vi "GOLPI Config Panel.vi"(8 "error in":errorcluster, 11 "session in":T2={"adc"={"niScope"={"channel cfg"=[], "sessions"=[], "multi cards"=FALSE, "channels"=0, "type"=enum."n/a", "memory [B/chn]"=0, "ext. clock [Hz]"=0.0, "samples count"=0, "use streaming"=FALSE, "proc setup"={"packet size [smpl]"=0, "current timeout [s]"=0.0, "blk2blk timeout [s]"=0.0, "event time"=timestamp(0 s since 1904-01-01), "temp sampl T [s]"=0.0, "data queue"=refnum, "stop notifier"=refnum, "proc ref"=refnum}, "sample width [B]"=0, "ranges [V]"=[], "trigger setup"={"coupling"=1, "level [V]"=0.0, "slope"=0, "mode"=enum."Immediate"}, "fs [Hz]"=0.0, "bitres [bit]"=0}, "3458A"={"channels"=[], "sync unit"={"VISA"="", "type"=enum."Picotest U6200A"}, "awg unit"={"type"=enum."Agilent 331xxA to 332xxA", "VISA"="", "enable 10MHz ref"=FALSE}, "sync mode"=enum."MASTER-SLAVE, MASTER clocked by TIMER", "streaming mode"=FALSE, "idn mode"=enum."Auto", "sampling mode"=enum."DCV", "Ts [s]"=0.0, "sample memory [B]"=0, "proc setup"={"channel id"=0, "packet size [smpl]"=0, "current timeout [s]"=0.0, "blk2blk timeout [s]"=0.0, "event time"=timestamp(0 s since 1904-01-01), "stop notifier"=refnum, "data queues"=[], "proc refs"=[], "bus semaphore"=refnum}, "sample size [B]"=0, "sample count"=0, "aux data"={"channel id"=0, "valid?"=[], "gain [V]"=[], "timestamp [s]"=[], "Ts [s]"=0.0, "abs timestamp"=timestamp(0 s since 1904-01-01), "t [deg C]"=[]}, "ranges [V]"=[], "aperture [s]"=0.0, "LEVEL trigger"={"edge"=enum."POS", "level [V]"=0.0, "coupling"=enum."DC"}, "trigger mode"=enum."AUTO", "measure temp.?"=FALSE, "disp mesages"=[], "shared bus?"=FALSE, "disable display?"=FALSE, "aper mode"=enum."Manual", "aper rules"=[]}, "dsdll"={"dsdll"={"dsdll path"=path "", "dsdll handle"=[], "output devices"=[], "capture devices"=[]}, "channels"=0, "device id"=0, "channel idns"=[], "proc setup"={"packet size [smpl]"=0, "current timeout [s]"=0.0, "blk2blk timeout [s]"=0.0, "event time"=timestamp(0 s since 1904-01-01), "data queue"=refnum, "stop notifier"=refnum, "proc ref"=refnum}, "samples count"=0, "fs [Hz]"=0.0}, "type"=enum."niScope", "channel idn str"=[], "aux instr idn str"=[], "modified?"=FALSE, "simadc"={"channels"=[], "range [V]"=0.0, "Ts step [s]"=0.0, "time [s]"=0.0, "fs [Hz]"=0.0, "count"=0, "smpl offset"=0, "set count"=0, "bit res"=0}, "force rst?"=FALSE, "exit mode"=enum."Immediate reset", "exit dly"=0.0, "exit tmr"=timestamp(0 s since 1904-01-01), "busy?"=FALSE, "accessed?"=FALSE, "QuADC session"={"channel cfg"=[], "sessions"=[], "multi cards"=FALSE, "channels"=0, "type"=enum."n/a", "memory [B/chn]"=0, "ext. clock [Hz]"=0.0, "samples count"=0, "use streaming"=FALSE, "proc setup"={"packet size [smpl]"=0, "current timeout [s]"=0.0, "blk2blk timeout [s]"=0.0, "event time"=timestamp(0 s since 1904-01-01), "temp sampl T [s]"=0.0, "data queue"=refnum, "stop notifier"=refnum, "proc ref"=refnum}, "sample width [B]"=0, "ranges [V]"=[], "trigger setup"={"coupling"=1, "level [V]"=0.0, "slope"=0, "mode"=enum."Immediate"}, "fs [Hz]"=0.0, "bitres [bit]"=0}}, "sequence"=[], "sequence setup"={"group setups"=[], "average cycles"=0, "range mode"=enum."Keep defaults", "fs mode"=enum."Frequency", "rng even"=0.0, "rng odd"=0.0, "folder"=path "", "name base"="", "meas id"=0, "settle [s]"=0.0}, "golpi"=refnum, "processing setup"={"mode"=enum."Raw", "call after avgs?"=FALSE, "calculate?"=FALSE, "raw mode"={"command"="", "result mode"=enum."Display console output (only Octave)", "res variable"=""}, "QWTB"={"QWTB path"=path "", "alg filter path"="", "alg ids"=[], "alg parameters"=[], "parsed parameters"=[], "selected alg id"="", "selected unc mode"=enum."None", "qwtb mcc"=100, "qwtb timeout"=90, "qwtb covg"=95.0, "qwtb ofs"=0, "qwtb lim data"=0, "multicore"={"jobs folder"=path "", "cores"=0, "max jobs"=0, "mode"=enum."Singlecore"}, "unc once?"=FALSE}}, "corrections"={"transducers"={"channels"=[], "last path"=path ""}, "digitizer"={"last path"=path "", "channel paths"=[], "channel idns"=[], "correction name"="", "channel names"=[], "folders to copy"=[], "channel valid"=[], "correction path"=path "", "correction rel path"="", "rel folders to copy"=[]}}, "assist cfg"={"P"=0, "Q"=0, "rel shift"=0.0, "ref freq"=0.0, "min fs"=0.0, "max fs tol"=0.0, "min int"=0.0, "max int"=0.0, "max err"=0.0, "max timeout"=0.0}} {"corrections"."transducers"."channels"."Phase index" min=1 step=1; "adc"."QuADC session"."trigger setup"."level [V]" format="%.2f"; "adc"."QuADC session"."trigger setup"."coupling" items=["AC"=0, "DC"=1, "HF Reject"=3, "LF Reject"=4, "AC Plus HF Reject"=1001]; "adc"."QuADC session"."channel cfg"."Clock fr. (Hz)" min=0.0 format="%#_9p"; "adc"."QuADC session"."channel cfg"."Number of JJ" min=1; "adc"."QuADC session"."channel cfg"."Range [Vpk]" min=0.0; "adc"."QuADC session"."channel cfg"."Channel" min=0; "adc"."3458A"."channels"."Range [Vpk]" min=0.0; "adc"."niScope"."trigger setup"."level [V]" format="%.2f"; "adc"."niScope"."trigger setup"."coupling" items=["AC"=0, "DC"=1, "HF Reject"=3, "LF Reject"=4, "AC Plus HF Reject"=1001]; "adc"."niScope"."channel cfg"."Range [Vpk]" min=0.0; "adc"."niScope"."channel cfg"."Channel" min=0}) -> (0 "error out":errorcluster, 3 "session out":T2={"adc"={"niScope"={"channel cfg"=[], "sessions"=[], "multi cards"=FALSE, "channels"=0, "type"=enum."n/a", "memory [B/chn]"=0, "ext. clock [Hz]"=0.0, "samples count"=0, "use streaming"=FALSE, "proc setup"={"packet size [smpl]"=0, "current timeout [s]"=0.0, "blk2blk timeout [s]"=0.0, "event time"=timestamp(0 s since 1904-01-01), "temp sampl T [s]"=0.0, "data queue"=refnum, "stop notifier"=refnum, "proc ref"=refnum}, "sample width [B]"=0, "ranges [V]"=[], "trigger setup"={"coupling"=1, "level [V]"=0.0, "slope"=0, "mode"=enum."Immediate"}, "fs [Hz]"=0.0, "bitres [bit]"=0}, "3458A"={"channels"=[], "sync unit"={"VISA"="", "type"=enum."Picotest U6200A"}, "awg unit"={"type"=enum."Agilent 331xxA to 332xxA", "VISA"="", "enable 10MHz ref"=FALSE}, "sync mode"=enum."MASTER-SLAVE, MASTER clocked by TIMER", "streaming mode"=FALSE, "idn mode"=enum."Auto", "sampling mode"=enum."DCV", "Ts [s]"=0.0, "sample memory [B]"=0, "proc setup"={"channel id"=0, "packet size [smpl]"=0, "current timeout [s]"=0.0, "blk2blk timeout [s]"=0.0, "event time"=timestamp(0 s since 1904-01-01), "stop notifier"=refnum, "data queues"=[], "proc refs"=[], "bus semaphore"=refnum}, "sample size [B]"=0, "sample count"=0, "aux data"={"channel id"=0, "valid?"=[], "gain [V]"=[], "timestamp [s]"=[], "Ts [s]"=0.0, "abs timestamp"=timestamp(0 s since 1904-01-01), "t [deg C]"=[]}, "ranges [V]"=[], "aperture [s]"=0.0, "LEVEL trigger"={"edge"=enum."POS", "level [V]"=0.0, "coupling"=enum."DC"}, "trigger mode"=enum."AUTO", "measure temp.?"=FALSE, "disp mesages"=[], "shared bus?"=FALSE, "disable display?"=FALSE, "aper mode"=enum."Manual", "aper rules"=[]}, "dsdll"={"dsdll"={"dsdll path"=path "", "dsdll handle"=[], "output devices"=[], "capture devices"=[]}, "channels"=0, "device id"=0, "channel idns"=[], "proc setup"={"packet size [smpl]"=0, "current timeout [s]"=0.0, "blk2blk timeout [s]"=0.0, "event time"=timestamp(0 s since 1904-01-01), "data queue"=refnum, "stop notifier"=refnum, "proc ref"=refnum}, "samples count"=0, "fs [Hz]"=0.0}, "type"=enum."niScope", "channel idn str"=[], "aux instr idn str"=[], "modified?"=FALSE, "simadc"={"channels"=[], "range [V]"=0.0, "Ts step [s]"=0.0, "time [s]"=0.0, "fs [Hz]"=0.0, "count"=0, "smpl offset"=0, "set count"=0, "bit res"=0}, "force rst?"=FALSE, "exit mode"=enum."Immediate reset", "exit dly"=0.0, "exit tmr"=timestamp(0 s since 1904-01-01), "busy?"=FALSE, "accessed?"=FALSE, "QuADC session"={"channel cfg"=[], "sessions"=[], "multi cards"=FALSE, "channels"=0, "type"=enum."n/a", "memory [B/chn]"=0, "ext. clock [Hz]"=0.0, "samples count"=0, "use streaming"=FALSE, "proc setup"={"packet size [smpl]"=0, "current timeout [s]"=0.0, "blk2blk timeout [s]"=0.0, "event time"=timestamp(0 s since 1904-01-01), "temp sampl T [s]"=0.0, "data queue"=refnum, "stop notifier"=refnum, "proc ref"=refnum}, "sample width [B]"=0, "ranges [V]"=[], "trigger setup"={"coupling"=1, "level [V]"=0.0, "slope"=0, "mode"=enum."Immediate"}, "fs [Hz]"=0.0, "bitres [bit]"=0}}, "sequence"=[], "sequence setup"={"group setups"=[], "average cycles"=0, "range mode"=enum."Keep defaults", "fs mode"=enum."Frequency", "rng even"=0.0, "rng odd"=0.0, "folder"=path "", "name base"="", "meas id"=0, "settle [s]"=0.0}, "golpi"=refnum, "processing setup"={"mode"=enum."Raw", "call after avgs?"=FALSE, "calculate?"=FALSE, "raw mode"={"command"="", "result mode"=enum."Display console output (only Octave)", "res variable"=""}, "QWTB"={"QWTB path"=path "", "alg filter path"="", "alg ids"=[], "alg parameters"=[], "parsed parameters"=[], "selected alg id"="", "selected unc mode"=enum."None", "qwtb mcc"=100, "qwtb timeout"=90, "qwtb covg"=95.0, "qwtb ofs"=0, "qwtb lim data"=0, "multicore"={"jobs folder"=path "", "cores"=0, "max jobs"=0, "mode"=enum."Singlecore"}, "unc once?"=FALSE}}, "corrections"={"transducers"={"channels"=[], "last path"=path ""}, "digitizer"={"last path"=path "", "channel paths"=[], "channel idns"=[], "correction name"="", "channel names"=[], "folders to copy"=[], "channel valid"=[], "correction path"=path "", "correction rel path"="", "rel folders to copy"=[]}}, "assist cfg"={"P"=0, "Q"=0, "rel shift"=0.0, "ref freq"=0.0, "min fs"=0.0, "max fs tol"=0.0, "min int"=0.0, "max int"=0.0, "max err"=0.0, "max timeout"=0.0}} {"corrections"."transducers"."channels"."Phase index" min=1 step=1; "adc"."QuADC session"."trigger setup"."level [V]" format="%.2f"; "adc"."QuADC session"."trigger setup"."coupling" items=["AC"=0, "DC"=1, "HF Reject"=3, "LF Reject"=4, "AC Plus HF Reject"=1001]; "adc"."QuADC session"."channel cfg"."Clock fr. (Hz)" min=0.0 format="%#_9p"; "adc"."QuADC session"."channel cfg"."Number of JJ" min=1; "adc"."QuADC session"."channel cfg"."Range [Vpk]" min=0.0; "adc"."QuADC session"."channel cfg"."Channel" min=0; "adc"."3458A"."channels"."Range [Vpk]" min=0.0; "adc"."niScope"."trigger setup"."level [V]" format="%.2f"; "adc"."niScope"."trigger setup"."coupling" items=["AC"=0, "DC"=1, "HF Reject"=3, "LF Reject"=4, "AC Plus HF Reject"=1001]; "adc"."niScope"."channel cfg"."Range [Vpk]" min=0.0; "adc"."niScope"."channel cfg"."Channel" min=0})   [LabVIEW 2018]
doc: "This is panel for configuration of Octave/Matlab interface."
uses:
  measure/Meas Session.ctl
  adc/ADC Session.ctl
  drivers/niScope/niScope Session.ctl
  drivers/niScope/niScope Virtual Channel Config.ctl
  drivers/niScope/niScope Virtual Channel Mode.ctl
  drivers/niScope/niScope Virtual Channel Input Z.ctl
  drivers/niScope/niScope Virtual Channel Coupling.ctl
  drivers/niScope/niScope Type.ctl
  drivers/niScope/niScope Digitizing Process Options.ctl
  drivers/niScope/niScope Data Packet.ctl
  drivers/niScope/niScope Trigger Setup.ctl
  <instrlib>/niScope/Controls/niScope trigger coupling.ctl
  <instrlib>/niScope/Controls/niScope trigger slope.ctl
  drivers/DMM/3458A Digitizer Session.ctl
  drivers/DMM/3458A Virtual Channel Config.ctl
  drivers/Counter/Counter Session.ctl
  drivers/Counter/Counter Type.ctl
  drivers/AWG/AWG Session.ctl
  drivers/AWG/AWG Type.ctl
  drivers/DMM/3458A Sync Mode.ctl
  drivers/DMM/3458A Idn Mode.ctl
  drivers/DMM/3458A Digitizing Low Levels/Configure/Sampling Mode.ctl
  drivers/DMM/3458A Digitizing Process Options.ctl
  drivers/DMM/3458A Data Packet.ctl
  drivers/DMM/3458A Aux Record Data.ctl
  drivers/DMM/3458A Digitizing Low Levels/Configure/Level Setup.ctl
  drivers/DMM/3458A Digitizing Low Levels/Configure/First Sample Trigger.ctl
  drivers/DMM/3458A Aperture Selection Mode.ctl
  drivers/dsdll/DSDLL Session.ctl
  drivers/dsdll/dsdll source distribution/dsdll_instance.ctl
  drivers/dsdll/dsdll source distribution/dsdll_device_record.ctl
  drivers/dsdll/DSDLL Process Config.ctl
  drivers/dsdll/DSDLL Data Packet.ctl
  adc/ADC Type.ctl
  drivers/simulated_adc/SimAdc Config.ctl
  drivers/simulated_adc/SimAdc Channel Cfg.ctl
  adc/ADC On Close Action.ctl
  drivers/Quatsch_driver/QuADCDriver/QuADC Session.ctl
  drivers/Quatsch_driver/QuADCDriver/QuADC Virtual Channel Config.ctl
  drivers/Quatsch_driver/QuADCDriver/QuADC Virtual Channel Mode.ctl
  drivers/Quatsch_driver/QuADCDriver/QuADC Virtual Channel Input Z.ctl
  drivers/Quatsch_driver/QuADCDriver/QuADC Virtual Channel Coupling.ctl
  drivers/Quatsch_driver/QuADCDriver/QuADC Type.ctl
  drivers/Quatsch_driver/QuADCDriver/QuADC Digitizing Process Options.ctl
  drivers/Quatsch_driver/QuADCDriver/QuADC Data Packet.ctl
  drivers/Quatsch_driver/QuADCDriver/QuADC Trigger Setup.ctl
  measure/Meas Sequence Item.ctl
  measure/Meas Sampling Configuration.ctl
  adc/ADC Trig Config.ctl
  adc/ADC Trig Mode Source.ctl
  adc/ADC Trig Coupling.ctl
  adc/ADC Trig Slope.ctl
  measure/processing/QWTB/Meas Proc QWTB Algorithm Parameter Data.ctl
  measure/Meas Sequence Configuration.ctl
  measure/Meas Range Mode.ctl
  measure/Meas Sampling Rate Mode.ctl
  golpi_session_ref.ctl
  golpi_session.ctl
  GOLPI Library.lvlibp/Public/GOLPI reference Type Def.ctl
  GOLPI Library.lvlibp/LV Process source distribution/Pipe Handle.ctl
  measure/processing/Meas Process Config.ctl
  measure/processing/Meas Process Mode.ctl
  measure/processing/Meas Process Raw Config.ctl
  measure/processing/Meas Process Raw Result Mode.ctl
  measure/processing/QWTB/Meas Proc QWTB Setup.ctl
  measure/processing/QWTB/Meas Proc QWTB Uncertainty Mode.ctl
  measure/processing/QWTB/Meas Proc QWTB Multicore Setup.ctl
  measure/processing/QWTB/Meas Proc QWTB Multicore Type.ctl
  measure/Corrections/Corr Setup.ctl
  measure/Corrections/Corr Tranducer Item.ctl
  measure/Corrections/Corr Digitizers.ctl
  measure/Assist/Assist Panel Setup.ctl
  varilib/SGUI Assign References Mode.ctl
  varilib/SGUI Assign Multiple Strings With Tags By Label.vi
  varilib/varilib.lvlib
  GOLPI Library.lvlibp
  GOLPI Multi Process.lvlib
  GOLPI Library.lvlibp/LV Process source distribution/LV Process library.lvlib
  drivers/niScope/niScope Virtual Digitizer.lvlib
  drivers/DMM/3458A Virtual Digitizer.lvlib
  drivers/Counter/Counter.lvlib
  drivers/AWG/AWG.lvlib
  drivers/DMM/3458A Digitizing Low Levels/3458A Digitizing Low Levels.lvlib
  drivers/dsdll/DSDLL Virtual Digitizer.lvlib
  drivers/Quatsch_driver/QuADCDriver/QuADC Virtual Digitizer.lvlib
  drivers/dsdll/dsdll source distribution/dsdll.lvlib
panel:
  out "golpi":T1
  in  "tc qwtb":enum32{"Page 1", "Page 2"}(tab)
  in  "qwtb filter":string caption="Relative path to the QWTB algorithms filter (list of supported algorithms)"
  out "qwtb status":bool
  in  "btn test qwtb":bool
  in  "qwtb path":path caption="QWTB toolbox root folder path"
  out "qwtb stat str":string caption="Status"
  in  "btn stop":bool
  in  "tc golpi stat":enum32{"Page 1", "Page 2"}(tab)
  out "status":bool
  out "ver":string caption="Octave version"
  in  "btn test":bool
  in  "btn ok":bool
  in  "tc main":enum32{"Page 1", "Page 2"}(tab)
  in  "btn matlab":bool caption="Enable Matlab Script mode"
  in  "btn clr cache":bool caption="Always clear function cache (slower)"
  in  "btn bitstream":bool caption="Use bitstream mode"
  out "golpi stat":bool caption="GOLPI/GNU Octave running?"
  in  "btn console":bool caption="Show console window"
  in  "start timeout [ms]":u32=30000 caption="Startup timeout [ms]"
  in  "octave path":path=path "C:/Octave/Octave_3.6.4/bin" caption="GNU Octave binary path (folder or full path)"
  # "Note: Restart GOLPI to apply changes!"
  # "ADC:"
  # "IP Address"
  # "."
  # "."
  # "."
  # ":"
  # "ADC:"
  # "IP Address"
  # "."
  # "."
  # "."
  # ":"
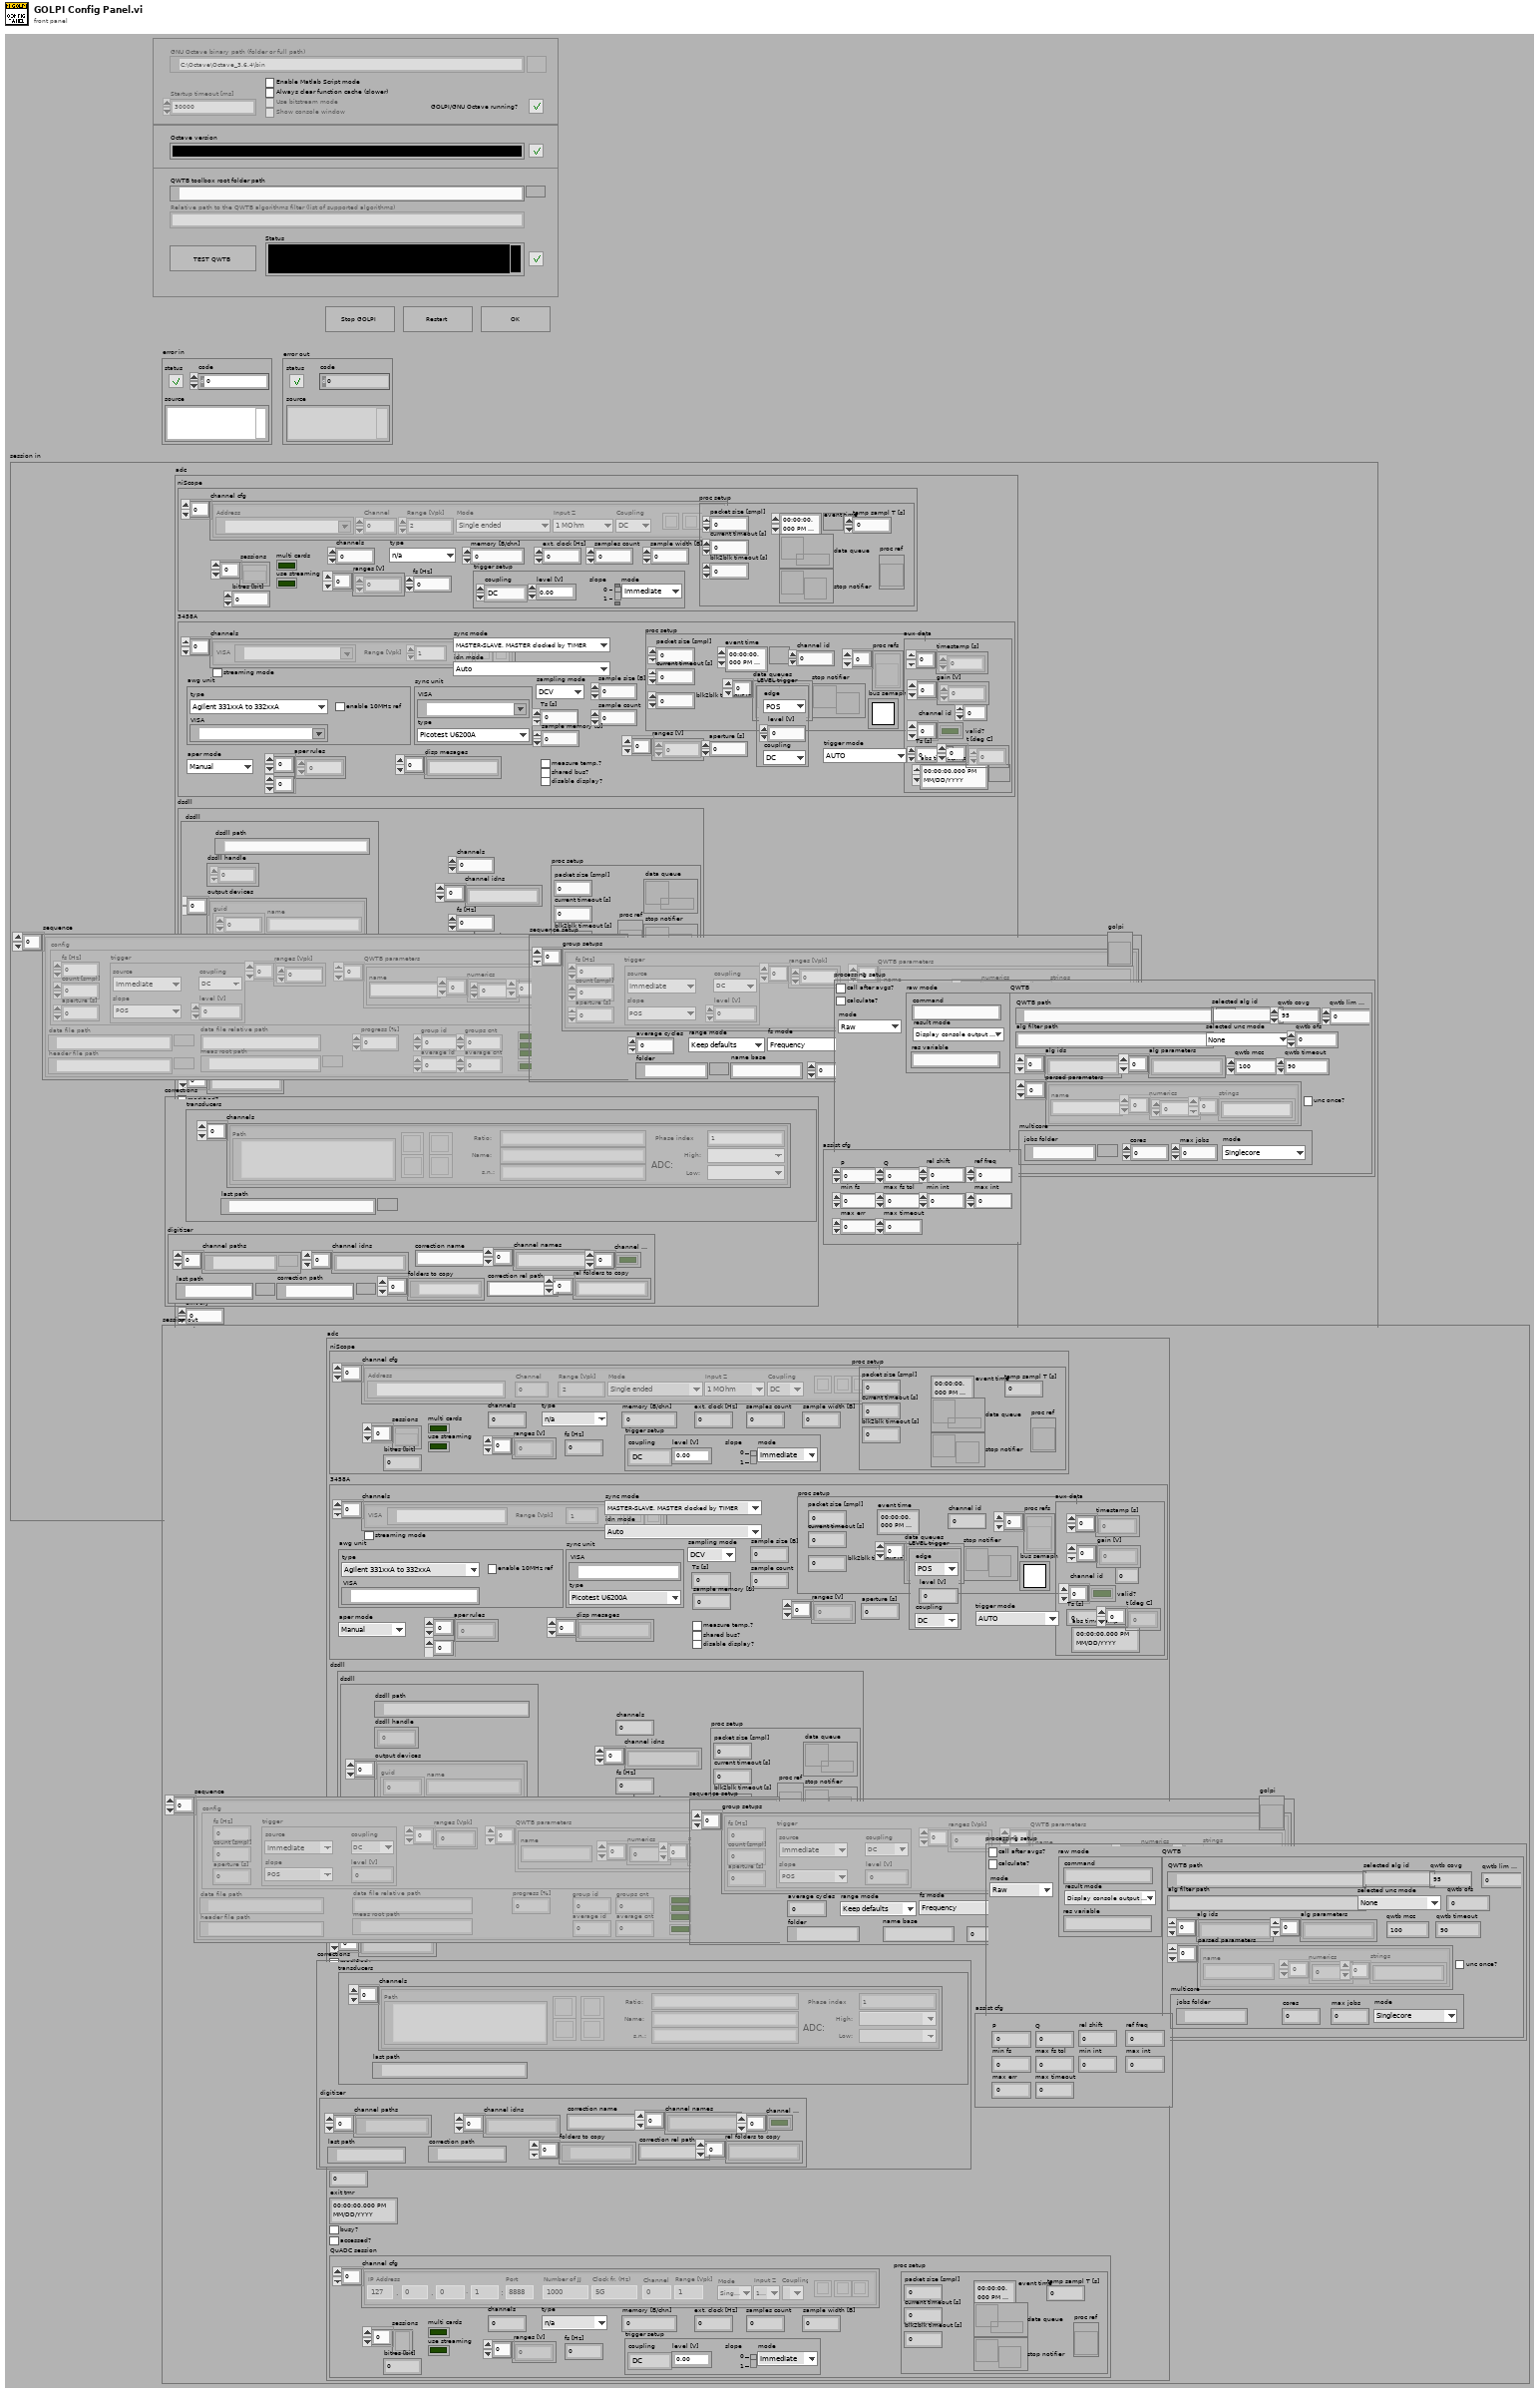
[diagram p1: front panel]
types:
  T1 = typedef "GOLPI Multi Process.lvlib/golpi_session_ref.ctl" = refnum<vi>
  T2 = typedef "Meas Session.ctl" = cluster{"adc":T3, "sequence":T45[], "sequence setup":T52, "golpi":T1, "processing setup":T55, "corrections":T63, "assist cfg":T66}
  T3 = typedef "ADC Session.ctl" = cluster{"niScope":T4, "3458A":T14, "dsdll":T29, "type":T33, "channel idn str":string[], "aux instr idn str":string[], "modified?":bool, "simadc":T34, "force rst?":bool, "exit mode":T36, "exit dly":dbl, "exit tmr":timestamp, "busy?":bool, "accessed?":bool, "QuADC session":T37}
  T4 = typedef "niScope Virtual Digitizer.lvlib/niScope Session.ctl" = cluster{"channel cfg":T5[], "sessions":refnum<k20>[], "multi cards":bool, "channels":i32, "type":T9, "memory [B/chn]":i32, "ext. clock [Hz]":dbl, "samples count":i64, "use streaming":bool, "proc setup":T10, "sample width [B]":i32, "ranges [V]":dbl[], "trigger setup":T11, "fs [Hz]":dbl, "bitres [bit]":i32}
  T5 = typedef "niScope Virtual Digitizer.lvlib/niScope Virtual Channel Config.ctl" = cluster{"Address":refnum<k15>, "Channel":i32, "Mode":T6, "Input Z":T7, "Coupling":T8, "Range [Vpk]":dbl, "btn clr":bool, "btn up":bool, "btn down":bool}
  T6 = typedef "niScope Virtual Digitizer.lvlib/niScope Virtual Channel Mode.ctl" = enum16{"Single ended", "Unbal. differential", "Differential"}
  T7 = typedef "niScope Virtual Digitizer.lvlib/niScope Virtual Channel Input Z.ctl" = enum16{"1 MOhm", "50 Ohm"}
  T8 = typedef "niScope Virtual Digitizer.lvlib/niScope Virtual Channel Coupling.ctl" = enum16{"AC", "DC", "GND"}
  T9 = typedef "niScope Virtual Digitizer.lvlib/niScope Type.ctl" = enum16{"n/a", "5922"}
  T10 = typedef "niScope Virtual Digitizer.lvlib/niScope Digitizing Process Options.ctl" = cluster{"packet size [smpl]":i64, "current timeout [s]":dbl, "blk2blk timeout [s]":dbl, "event time":timestamp, "temp sampl T [s]":dbl, "data queue":refnum<queue>, "stop notifier":refnum<notifier>, "proc ref":refnum<vi>}
  T11 = typedef "niScope Virtual Digitizer.lvlib/niScope Trigger Setup.ctl" = cluster{"coupling":T12, "level [V]":dbl, "slope":T13, "mode":enum16{"Immediate", "External", "Level"}}
  T12 = typedef "niScope trigger coupling.ctl" = u16
  T13 = typedef "niScope trigger slope.ctl" = i32
  T14 = typedef "3458A Virtual Digitizer.lvlib/3458A Digitizer Session.ctl" = cluster{"channels":T15[], "sync unit":T16, "awg unit":T18, "sync mode":T20, "streaming mode":bool, "idn mode":T21, "sampling mode":T22, "Ts [s]":dbl, "sample memory [B]":i32, "proc setup":T23, "sample size [B]":i32, "sample count":i32, "aux data":T25, "ranges [V]":dbl[], "aperture [s]":dbl, "LEVEL trigger":T26, "trigger mode":T27, "measure temp.?":bool, "disp mesages":string[], "shared bus?":bool, "disable display?":bool, "aper mode":T28, "aper rules":dbl[][]}
  T15 = typedef "3458A Virtual Digitizer.lvlib/3458A Virtual Channel Config.ctl" = cluster{"VISA":refnum<visa-resource-name>, "Range [Vpk]":dbl, "btn clr":bool, "btn up":bool, "btn down":bool}
  T16 = typedef "Counter.lvlib/Counter Session.ctl" = cluster{"VISA":refnum<visa-resource-name>, "type":T17}
  T17 = typedef "Counter.lvlib/Counter Type.ctl" = enum16{"Picotest U6200A", "dummy"}
  T18 = typedef "AWG.lvlib/AWG Session.ctl" = cluster{"type":T19, "VISA":refnum<visa-resource-name>, "enable 10MHz ref":bool}
  T19 = typedef "AWG.lvlib/AWG Type.ctl" = enum16{"Agilent 331xxA to 332xxA", "Agilent 335xxA to 336xxA", "Tektronix AFG3101C", "dummy"}
  T20 = typedef "3458A Virtual Digitizer.lvlib/3458A Sync Mode.ctl" = enum16{"MASTER-SLAVE, MASTER clocked by TIMER", "MASTER-SLAVE, MASTER clocked by AWG", "ALL clocked by AWG", "MASTER-SLAVE, ALL clocked by TIMER", "ALL clocked by AWG with DFLL"}
  T21 = typedef "3458A Virtual Digitizer.lvlib/3458A Idn Mode.ctl" = enum16{"Auto", "Sequential (chn A, chn B, ...)", "From calibration string"}
  T22 = typedef "3458A Virtual Digitizer.lvlib/3458A Digitizing Low Levels.lvlib/Sampling Mode.ctl" = enum16{"DCV", "DSDC", "DSAC"}
  T23 = typedef "3458A Virtual Digitizer.lvlib/3458A Digitizing Process Options.ctl" = cluster{"channel id":i32, "packet size [smpl]":i32, "current timeout [s]":dbl, "blk2blk timeout [s]":dbl, "event time":timestamp, "stop notifier":refnum<notifier>, "data queues":refnum<queue>[], "proc refs":refnum<vi>[], "bus semaphore":T24}
  T24 = typedef "Semaphore RefNum" = refnum<k1>
  T25 = typedef "3458A Virtual Digitizer.lvlib/3458A Aux Record Data.ctl" = cluster{"channel id":i32, "valid?":bool[], "gain [V]":dbl[], "timestamp [s]":dbl[], "Ts [s]":dbl, "abs timestamp":timestamp, "t [deg C]":dbl[]}
  T26 = typedef "3458A Virtual Digitizer.lvlib/3458A Digitizing Low Levels.lvlib/Level Setup.ctl" = cluster{"edge":enum16{"POS", "NEG"}, "level [V]":dbl, "coupling":enum16{"DC", "AC"}}
  T27 = typedef "3458A Virtual Digitizer.lvlib/3458A Digitizing Low Levels.lvlib/First Sample Trigger.ctl" = enum16{"AUTO", "EXT", "SYN", "SGL", "HOLD", "LEVEL"}
  T28 = typedef "3458A Virtual Digitizer.lvlib/3458A Aperture Selection Mode.ctl" = enum16{"Manual", "Maximum", "Table"}
  T29 = typedef "DSDLL Virtual Digitizer.lvlib/DSDLL Session.ctl" = cluster{"dsdll":T30, "channels":i32, "device id":i32, "channel idns":string[], "proc setup":T32, "samples count":i32, "fs [Hz]":dbl}
  T30 = typedef "dsdll.lvlib/dsdll_instance.ctl" = cluster{"dsdll path":path, "dsdll handle":u8[], "output devices":T31[], "capture devices":T31[]}
  T31 = typedef "dsdll.lvlib/dsdll_device_record.ctl" = cluster{"guid":u8[], "name":string}
  T32 = typedef "DSDLL Virtual Digitizer.lvlib/DSDLL Process Config.ctl" = cluster{"packet size [smpl]":i32, "current timeout [s]":dbl, "blk2blk timeout [s]":dbl, "event time":timestamp, "data queue":refnum<queue>, "stop notifier":refnum<notifier>, "proc ref":refnum<vi>}
  T33 = typedef "ADC Type.ctl" = enum16{"niScope", "3458A", "DirectSound DLL", "dummy", "QuADC"}
  T34 = typedef "SimAdc Config.ctl" = cluster{"channels":T35[], "range [V]":dbl, "Ts step [s]":dbl, "time [s]":dbl, "fs [Hz]":dbl, "count":i64, "smpl offset":i64, "set count":i64, "bit res":i32}
  T35 = typedef "SimAdc Channel Cfg.ctl" = cluster{"harmonics":dbl[][], "btn clear":bool, "noise":dbl, "fundamental [Hz]":dbl}
  T36 = typedef "ADC On Close Action.ctl" = enum16{"Immediate reset", "Delayed reset"}
  T37 = typedef "QuADC Virtual Digitizer.lvlib/QuADC Session.ctl" = cluster{"channel cfg":T38[], "sessions":refnum<k5>[], "multi cards":bool, "channels":i32, "type":T42, "memory [B/chn]":i32, "ext. clock [Hz]":dbl, "samples count":i64, "use streaming":bool, "proc setup":T43, "sample width [B]":i32, "ranges [V]":dbl[], "trigger setup":T44, "fs [Hz]":dbl, "bitres [bit]":i32}
  T38 = typedef "QuADC Virtual Digitizer.lvlib/QuADC Virtual Channel Config.ctl" = cluster{"Channel":i32, "Mode":T39, "Input Z":T40, "Coupling":T41, "Range [Vpk]":dbl, "btn clr":bool, "btn up":bool, "btn down":bool, "IP address A":u8, "IP address B":u8, "IP address C":u8, "IP address D":u8, "Port":u16, "Number of JJ":u32, "Clock fr. (Hz)":dbl}
  T39 = typedef "QuADC Virtual Digitizer.lvlib/QuADC Virtual Channel Mode.ctl" = enum16{"Single ended", "Unbal. differential", "Differential"}
  T40 = typedef "QuADC Virtual Digitizer.lvlib/QuADC Virtual Channel Input Z.ctl" = enum16{"1 MOhm", "50 Ohm"}
  T41 = typedef "QuADC Virtual Digitizer.lvlib/QuADC Virtual Channel Coupling.ctl" = enum16{"AC", "DC", "GND"}
  T42 = typedef "QuADC Virtual Digitizer.lvlib/QuADC Type.ctl" = enum16{"n/a", "v1"}
  T43 = typedef "QuADC Virtual Digitizer.lvlib/QuADC Digitizing Process Options.ctl" = cluster{"packet size [smpl]":i64, "current timeout [s]":dbl, "blk2blk timeout [s]":dbl, "event time":timestamp, "temp sampl T [s]":dbl, "data queue":refnum<queue>, "stop notifier":refnum<notifier>, "proc ref":refnum<vi>}
  T44 = typedef "QuADC Virtual Digitizer.lvlib/QuADC Trigger Setup.ctl" = cluster{"coupling":T12, "level [V]":dbl, "slope":T13, "mode":enum16{"Immediate", "External", "Level"}}
  T45 = typedef "Meas Sequence Item.ctl" = cluster{"config":T46, "data file path":path, "header file path":path, "group id":i32, "average id":i32, "group done?":bool, "adc modified?":bool, "source modified?":bool, "progress [%]":dbl, "groups cnt":i32, "average cnt":i32, "data file relative path":string, "meas root path":path, "calculate?":bool}
  T46 = typedef "Meas Sampling Configuration.ctl" = cluster{"fs [Hz]":dbl, "count [smpl]":i64, "aperture [s]":dbl, "trigger":T47, "ranges [Vpk]":dbl[], "QWTB parameters":T51[]}
  T47 = typedef "ADC Trig Config.ctl" = cluster{"source":T48, "level [V]":dbl, "coupling":T49, "slope":T50}
  T48 = typedef "ADC Trig Mode Source.ctl" = enum16{"Immediate", "External", "Level"}
  T49 = typedef "ADC Trig Coupling.ctl" = enum16{"DC", "AC"}
  T50 = typedef "ADC Trig Slope.ctl" = enum16{"POS", "NEG"}
  T51 = typedef "Meas Proc QWTB Algorithm Parameter Data.ctl" = cluster{"name":string, "numerics":dbl[], "strings":string[]}
  T52 = typedef "Meas Sequence Configuration.ctl" = cluster{"group setups":T46[], "average cycles":i32, "range mode":T53, "fs mode":T54, "rng even":dbl, "rng odd":dbl, "folder":path, "name base":string, "meas id":i32, "settle [s]":dbl}
  T53 = typedef "Meas Range Mode.ctl" = enum16{"Keep defaults", "Set All channels", "Set Odd and Even channels"}
  T54 = typedef "Meas Sampling Rate Mode.ctl" = enum16{"Frequency", "Period"}
  T55 = typedef "Meas Process Config.ctl" = cluster{"mode":T56, "call after avgs?":bool, "calculate?":bool, "raw mode":T57, "QWTB":T59}
  T56 = typedef "Meas Process Mode.ctl" = enum16{"Raw", "QWTB"}
  T57 = typedef "Meas Process Raw Config.ctl" = cluster{"command":string, "result mode":T58, "res variable":string}
  T58 = typedef "Meas Process Raw Result Mode.ctl" = enum16{"Display console output (only Octave)", "Display string variable", "Display result file %respath%"}
  T59 = typedef "Meas Proc QWTB Setup.ctl" = cluster{"QWTB path":path, "alg filter path":string, "alg ids":string[], "alg parameters":string[], "parsed parameters":T51[], "selected alg id":string, "selected unc mode":T60, "qwtb mcc":i32, "qwtb timeout":i32, "qwtb covg":dbl, "qwtb ofs":i64, "qwtb lim data":i64, "multicore":T61, "unc once?":bool}
  T60 = typedef "Meas Proc QWTB Uncertainty Mode.ctl" = enum16{"None", "GUF", "Monte Carlo"}
  T61 = typedef "Meas Proc QWTB Multicore Setup.ctl" = cluster{"jobs folder":path, "cores":i32, "max jobs":i32, "mode":T62}
  T62 = typedef "Meas Proc QWTB Multicore Type.ctl" = enum16{"Singlecore", "Multicore", "Multistation"}
  T63 = typedef "Corr Setup.ctl" = cluster{"transducers":cluster{"channels":T64[], "last path":path}, "digitizer":T65}
  T64 = typedef "Corr Tranducer Item.ctl" = cluster{"Path":path, "Ratio:":string, "Name:":string, "btn rem":bool, "btn up":bool, "btn down":bool, "s.n.:":string, "btn open":bool, "ratio o/i":dbl, "chn hi":u16, "chn lo":u16, "Phase index":i32}
  T65 = typedef "Corr Digitizers.ctl" = cluster{"last path":path, "channel paths":path[], "channel idns":string[], "correction name":string, "channel names":string[], "folders to copy":path[], "channel valid":bool[], "correction path":path, "correction rel path":string, "rel folders to copy":string[]}
  T66 = typedef "Assist Panel Setup.ctl" = cluster{"P":i32, "Q":i32, "rel shift":dbl, "ref freq":dbl, "min fs":dbl, "max fs tol":dbl, "min int":dbl, "max int":dbl, "max err":dbl, "max timeout":dbl}
  T67 = typedef "varilib.lvlib/SGUI Assign References Mode.ctl" = enum16{"Add to stack", "Overwrite", "Release last", "Release ID"}
  T68 = typedef "GOLPI Library.lvlibp/GOLPI reference Type Def.ctl" = cluster{"pipe handle":T69, "fast read timeout [ms]":u32, "fast read settle time [ms]":u32, "fast read to multiple [ms]":u32, "max elements per input line":u32, "slow read timeout [ms]":u32, "stdin double format specifier":string, "max elements per stdout output column":u32, "console mode bitstream":bool, "bitstream first read timeout [ms]":u32, "bitstream read timeout [ms]":u32, "struct transfer possible":bool, "matlab mode":bool}
  T69 = typedef "GOLPI Library.lvlibp/LV Process library.lvlib/Pipe Handle.ctl" = cluster{"lv_proc.dll file path":path, "process instance handle":u32[], "debug mode":bool, "debug data":cluster{"time":timestamp, "stdin":bool, "data":string}[]}
  T70 = typedef "GOLPI Multi Process.lvlib/golpi_session.ctl" = cluster{"GOLPI ref":T68, "idn str":string, "octave path":path, "work path":path, "start timeout [ms]":u32, "clr cache":bool, "console":bool, "binary":bool, "semaphore":T24, "initial command":string, "exit command":string, "matlab":bool}
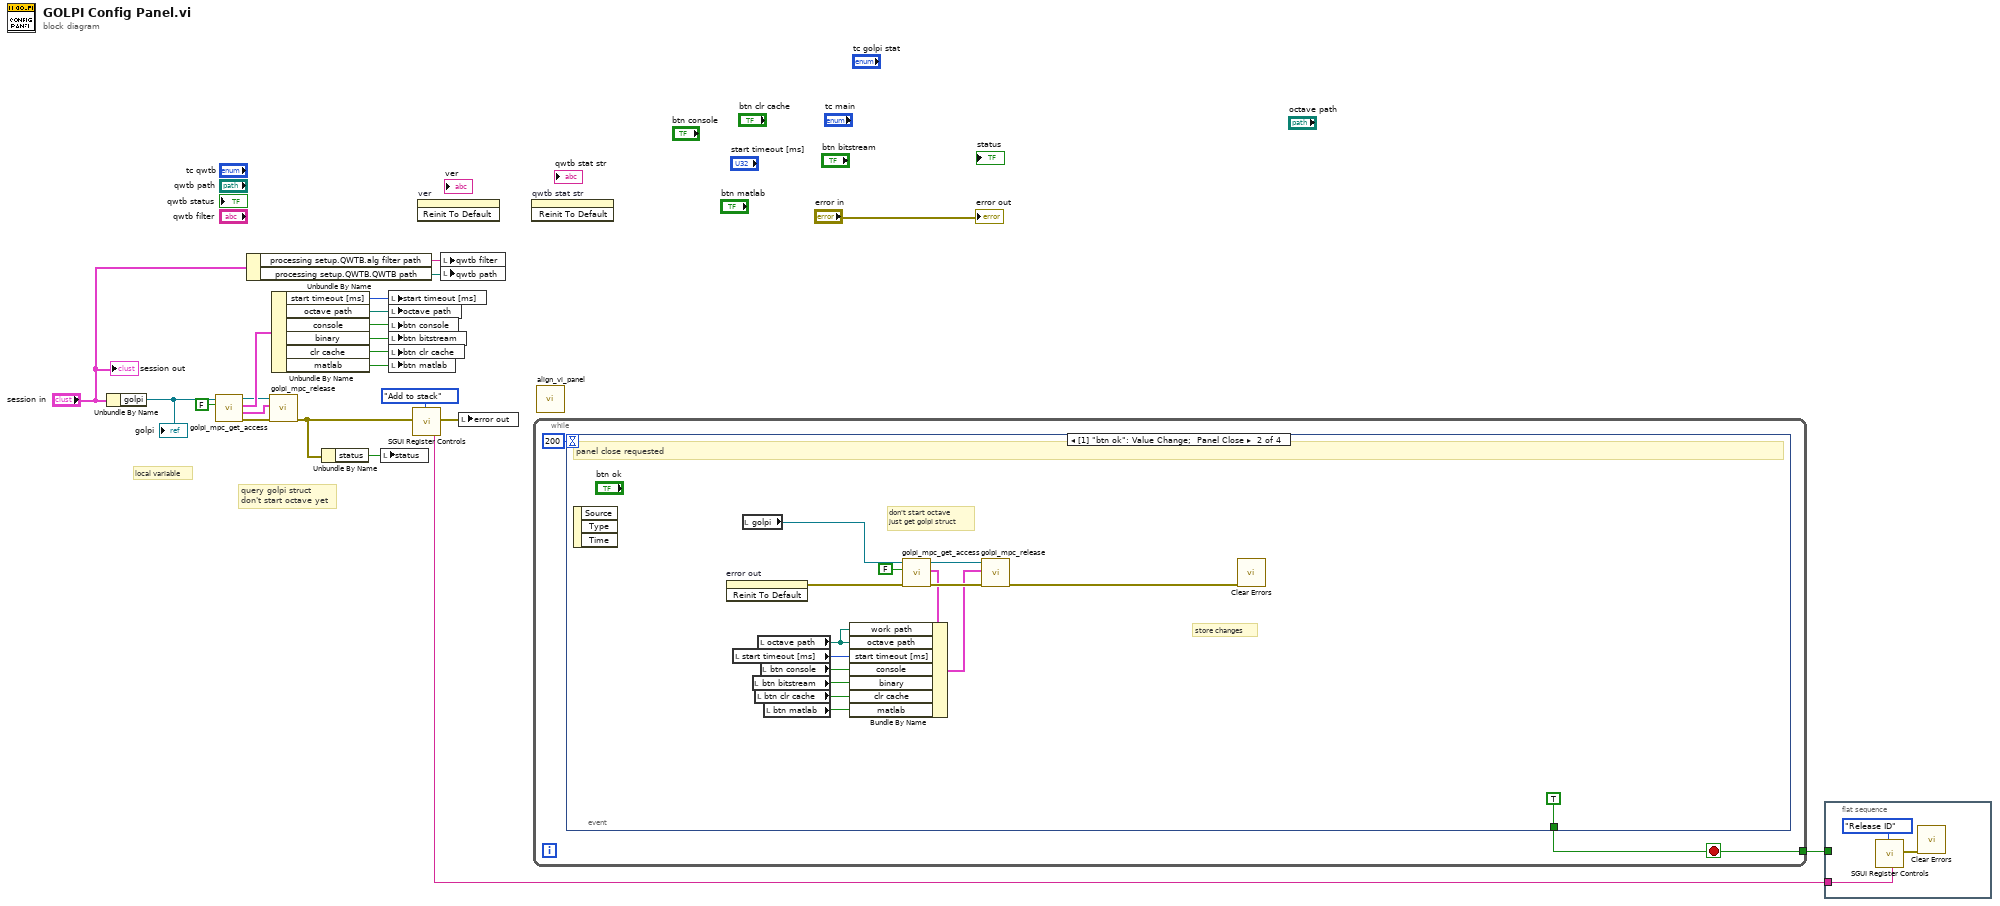
[diagram p0: block diagram]
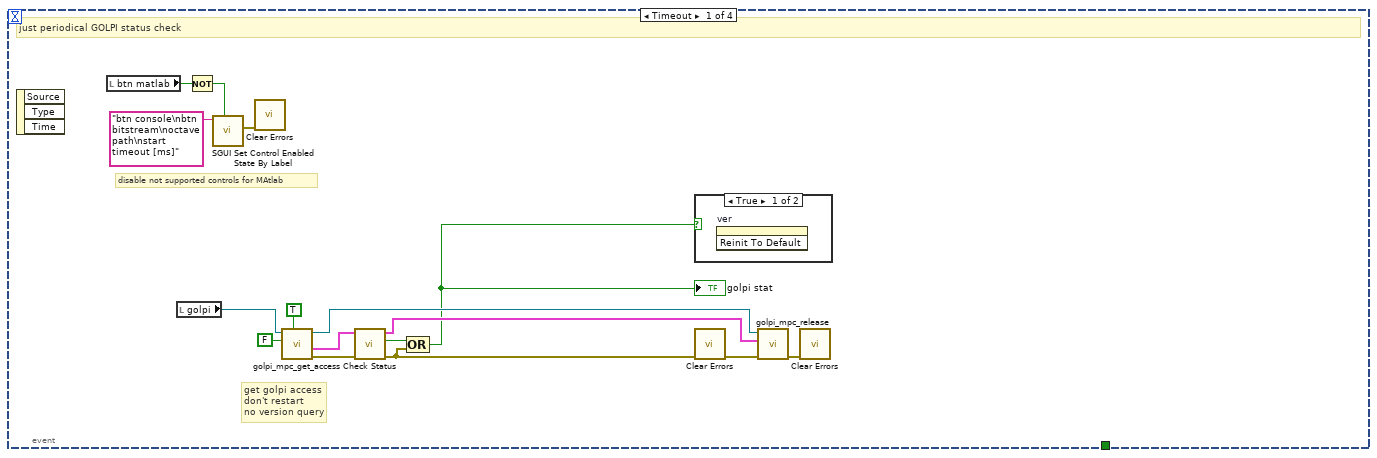
[diagram p2: hidden frame]
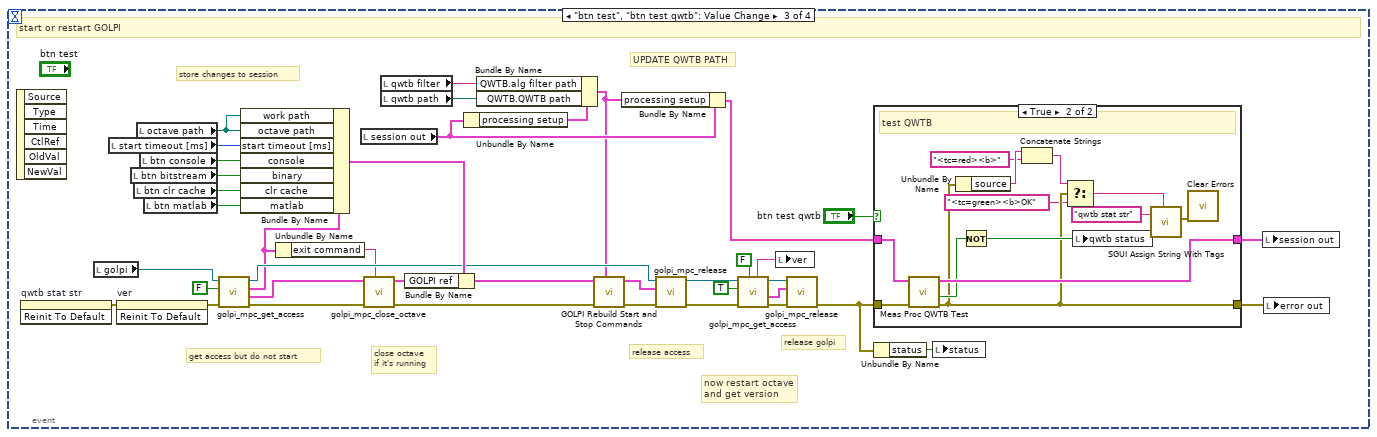
[diagram p4: hidden frame]
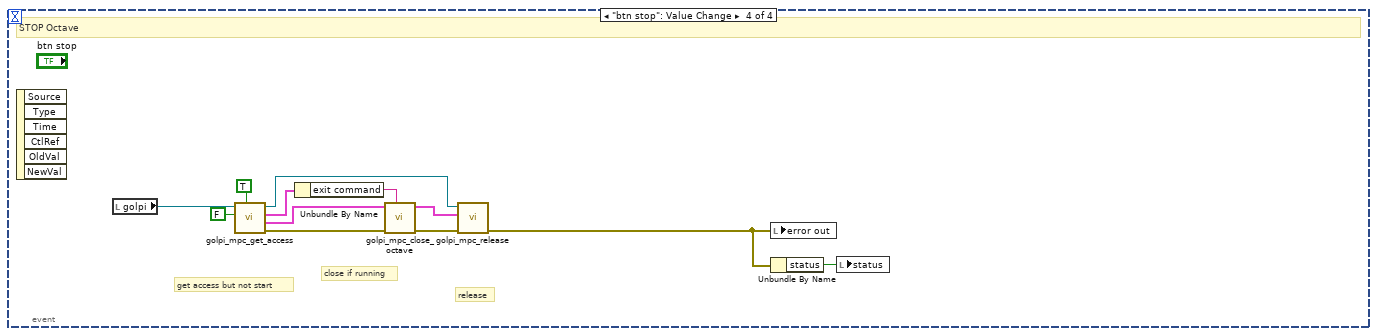
[diagram p6: hidden frame]
diagram:
  # "local variable"
  # "query golpi struct\ndon't start octave yet"
  n1 = Unbundle By Name("session in") -> ("golpi"=w10:T1)
  "golpi" <- w10
  n2 = call "golpi_mpc_get_access.vi"("allow octave start (true)"=FALSE, "golpi session ref"=w10) -> ("error out"=w17:errorcluster, "GOLPI ref out"=w14:T68, "golpi session out"=w16:T70, "golpi session ref out (copy)"=w15:T1)  [unwired: 4 in, 2 out]
  n3 = Unbundle By Name("session in") -> ("processing setup.QWTB.alg filter path"=w7:string, "processing setup.QWTB.QWTB path"=w8:path)
  n4 = call "golpi_mpc_release.vi"("error in"=w17, "golpi ref or golpi session in"=w14, "golpi session ref"=w15) -> ("error out"=w6:errorcluster)  [unwired: 7 in, 1 out]
  n5 = Unbundle By Name(w16) -> ("start timeout [ms]"=w21:u32, "octave path"=w20:path, "console"=w19:bool, "binary"=w12:bool, "clr cache"=w11:bool, "matlab"=w2:bool)
  n6 = Unbundle By Name(w6) -> ("status"=w18:bool)
  n7 = local write "status"(w18) -> ()
  n8 = local write "start timeout [ms]"(w21) -> ()
  n9 = local write "octave path"(w20) -> ()
  n10 = local write "btn console"(w19) -> ()
  n11 = local write "btn bitstream"(w12) -> ()
  n12 = local write "btn clr cache"(w11) -> ()
  n13 = local write "btn matlab"(w2) -> ()
  n14 = call "SGUI Register Controls.vi"("error in"=w6, "register mode (overwrite)"=SGUI_Assign_References_Mode."Add to stack") -> ("assigned ID"=w1:string, "error out"=w5:errorcluster)  [unwired: 15 in, 1 out]
  n15 = invoke on="ver" class="Str" method="Reinit To Default"() -> ()  [unwired: 3 in, 3 out]
  n16 = local write "qwtb filter"(w7) -> ()
  n17 = local write "qwtb path"(w8) -> ()
  n18 = local write "error out"(w5) -> ()
  n19 = invoke on="qwtb stat str" class="Str" method="Reinit To Default"() -> ()  [unwired: 3 in, 3 out]
  n20 = while {
    tunnel: [w23] -> w3
    stop <- w23 stop-if-true
    n21 = event shown="[1] \"btn ok\": Value Change;  Panel Close" {
      selector: _ -> [_ _ _ _]
      dyn-events: _ -> [_ _ _ _]
      timeout: 200 -> [_ _ _ _]
      tunnel: [_ TRUE _ _] -> w23
      event Timeout {
        # "disable not supported controls for MAtlab"
        # "get golpi access\ndon't restart\nno version query"
        # "just periodical GOLPI status check"
        n22 = event-data() -> ()  [unwired: 1 in, 3 out]
        n23 = local read "btn matlab"() -> (w28:bool)
        n24 = local read "golpi"() -> (w37:T1)
        n25 = Not(x=w28) -> (.not. x?=w26:bool)
        n26 = call "SGUI Set Control Enabled State By Label.vi"("labels (empty)"="btn console\nbtn bitstream\noctave path\nstart timeout [ms]", "Enabled? (False)"=w26) -> ("error out"=w25:errorcluster)  [unwired: 8 in, 1 out]
        n27 = call <vilib>:"Clear Errors.vi"("error in (no error)"=w25) -> ()  [unwired: 5 in, 2 out]
        n28 = call "golpi_mpc_get_access.vi"("don't query version (true)"=TRUE, "allow octave start (true)"=FALSE, "golpi session ref"=w37) -> ("error out"=w40:errorcluster, "GOLPI ref out"=w39:T68, "golpi session ref out (copy)"=w35:T1)  [unwired: 3 in, 3 out]
        n29 = call "Check Status.vi"("error in"=w40, "GOLPI ref. in"=w39) -> ("error out"=w32:errorcluster, "exited?"=w31:bool, "GOLPI ref. out"=w34:T68)  [unwired: 7 in]
        n30 = Compound Arithmetic op=OR(w31, w32) -> (w30:bool)
        "golpi stat" <- w30
        n31 = case shown="True" w30 {
          frame True {
            n32 = invoke on="ver" class="Str" method="Reinit To Default"() -> ()  [unwired: 3 in, 3 out]
          }
          frame False {
          }
        }
        n33 = call <vilib>:"Clear Errors.vi"("error in (no error)"=w32) -> ("error out"=w36:errorcluster)  [unwired: 5 in, 1 out]
        n34 = call "golpi_mpc_release.vi"("error in"=w36, "golpi ref or golpi session in"=w34, "golpi session ref"=w35) -> ("error out"=w29:errorcluster)  [unwired: 7 in, 1 out]
        n35 = call <vilib>:"Clear Errors.vi"("error in (no error)"=w29) -> ()  [unwired: 5 in, 2 out]
      }
      event "btn ok": Value Change; Panel Close {
        # "store changes"
        # "don't start octave\njust get golpi struct"
        # "panel close requested"
        n36 = event-data() -> ()  [unwired: 1 in, 3 out]
        n37 = invoke on="error out" class="Clust (strict)" method="Reinit To Default"() -> (error out=w42:errorcluster)  [unwired: 3 in, 2 out]
        n38 = local read "start timeout [ms]"() -> (w54:u32)
        n39 = local read "golpi"() -> (w49:T1)
        n40 = local read "btn bitstream"() -> (w44:bool)
        n41 = local read "btn clr cache"() -> (w43:bool)
        n42 = local read "octave path"() -> (w52:path)
        n43 = local read "btn console"() -> (w53:bool)
        n44 = local read "btn matlab"() -> (w41:bool)
        n45 = call "golpi_mpc_get_access.vi"("error in"=w42, "allow octave start (true)"=FALSE, "golpi session ref"=w49) -> ("error out"=w51:errorcluster, "golpi session out"=w48:T70, "golpi session ref out (copy)"=w50:T1)  [unwired: 3 in, 3 out]
        n46 = Bundle By Name(cluster=w48, "work path"=w52, "octave path"=w52, "start timeout [ms]"=w54, "console"=w53, "binary"=w44, "clr cache"=w43, "matlab"=w41) -> (w47:T70)
        n47 = call "golpi_mpc_release.vi"("error in"=w51, "golpi ref or golpi session in"=w47, "golpi session ref"=w50) -> ("error out"=w46:errorcluster)  [unwired: 7 in, 1 out]
        n48 = call <vilib>:"Clear Errors.vi"("error in (no error)"=w46) -> ()  [unwired: 5 in, 2 out]
      }
      event "btn test", "btn test qwtb": Value Change {
        # "UPDATE QWTB PATH"
        # "get access but do not start"
        # "store changes to session"
        # "release golpi"
        # "now restart octave\nand get version"
        # "release access"
        # "close octave\nif it's running"
        # "start or restart GOLPI"
        n49 = event-data() -> ()  [unwired: 1 in, 6 out]
        n50 = invoke on="qwtb stat str" class="Str" method="Reinit To Default"() -> (error out=w60:errorcluster)  [unwired: 3 in, 2 out]
        n51 = local read "golpi"() -> (w80:T1)
        n52 = local read "start timeout [ms]"() -> (w94:u32)
        n53 = invoke on="ver" class="Str" method="Reinit To Default"(error in=w60) -> (error out=w82:errorcluster)  [unwired: 2 in, 2 out]
        n54 = local read "btn bitstream"() -> (w84:bool)
        n55 = local read "btn clr cache"() -> (w83:bool)
        n56 = local read "octave path"() -> (w92:path)
        n57 = local read "btn console"() -> (w93:bool)
        n58 = local read "btn matlab"() -> (w56:bool)
        n59 = call "golpi_mpc_get_access.vi"("error in"=w82, "allow octave start (true)"=FALSE, "golpi session ref"=w80) -> ("error out"=w81:errorcluster, "GOLPI ref out"=w78:T68, "golpi session out"=w73:T70, "golpi session ref out (copy)"=w74:T1)  [unwired: 3 in, 2 out]
        n60 = Bundle By Name(cluster=w73, "work path"=w92, "octave path"=w92, "start timeout [ms]"=w94, "console"=w93, "binary"=w84, "clr cache"=w83, "matlab"=w56) -> (w77:T70)
        n61 = Unbundle By Name(w73) -> ("exit command"=w72:string)
        n62 = local read "session out"() -> (w66:T2)
        n63 = call "golpi_mpc_close_octave.vi"("exit command (empty)"=w72, "error in"=w81, "GOLPI ref in"=w78) -> ("error out"=w71:errorcluster, "GOLPI ref out (empty)"=w76:T68)  [unwired: 6 in, 1 out]
        n64 = local read "qwtb filter"() -> (w57:string)
        n65 = local read "qwtb path"() -> (w58:path)
        n66 = Bundle By Name(cluster=w77, "GOLPI ref"=w76) -> (w70:T70)
        n67 = Unbundle By Name(w66) -> ("processing setup"=w67:T55)
        n68 = Bundle By Name(cluster=w67, "QWTB.alg filter path"=w57, "QWTB.QWTB path"=w58) -> (w65:T55)
        n69 = call "GOLPI Rebuild Start and Stop Commands.vi"("processing setup"=w65, "error in"=w71, "golpi session in"=w70) -> ("error out"=w69:errorcluster, "golpi session out"=w68:T70)  [unwired: 7 in]
        n70 = Bundle By Name(cluster=w66, "processing setup"=w65) -> (w63:T2)
        n71 = call "golpi_mpc_release.vi"("error in"=w69, "golpi ref or golpi session in"=w68, "golpi session ref"=w74) -> ("error out"=w91:errorcluster, "golpi session out (copy)"=w90:T1)  [unwired: 7 in]
        n72 = call "golpi_mpc_get_access.vi"("don't query version (true)"=FALSE, "error in"=w91, "allow octave start (true)"=TRUE, "golpi session ref"=w90) -> ("error out"=w88:errorcluster, "GOLPI ref out"=w86:T68, "golpi session ref out (copy)"=w87:T1, "GNU Octave version"=w85:string)  [unwired: 2 in, 2 out]
        n73 = local write "ver"(w85) -> ()
        n74 = call "golpi_mpc_release.vi"("error in"=w88, "golpi ref or golpi session in"=w86, "golpi session ref"=w87) -> ("error out"=w59:errorcluster)  [unwired: 7 in, 1 out]
        n75 = case shown="True" "btn test qwtb" {
          tunnel: w59 -> [w96 w110]
          tunnel: [w96 w105] -> w64
          tunnel: w63 -> [w97 w109]
          tunnel: [w97 w108] -> w61
          frame False {
          }
          frame True {
            # "test QWTB"
            n76 = call "Meas Proc QWTB Test.vi"("error in"=w110, "session in"=w109) -> ("error out"=w105:errorcluster, "ok?"=w107:bool, "session out"=w108:T2)  [unwired: 7 in]
            n77 = Unbundle By Name(w105) -> ("source"=w103:string)
            n78 = Not(x=w107) -> (.not. x?=w106:bool)
            n79 = Concatenate Strings(w103, "<tc=red><b>" ("string")) -> (w102:string)
            n80 = Select(t=w102, s=w105, f="<tc=green><b>OK") -> (s? t:f=w100:string)
            n81 = local write "qwtb status"(w106) -> ()
            n82 = call-poly "SGUI Assign String With Tags.vi"("label(s) (empty)"="qwtb stat str", "string (empty)"=w100) -> ("error out"=w98:errorcluster)  [unwired: 8 in, 1 out]
            n83 = call <vilib>:"Clear Errors.vi"("error in (no error)"=w98) -> ()  [unwired: 5 in, 2 out]
          }
        }
        n84 = Unbundle By Name(w59) -> ("status"=w95:bool)
        n85 = local write "status"(w95) -> ()
        n86 = local write "session out"(w61) -> ()
        n87 = local write "error out"(w64) -> ()
      }
      event "btn stop": Value Change {
        # "release"
        # "close if running"
        # "get access but not start"
        # "STOP Octave"
        n88 = event-data() -> ()  [unwired: 1 in, 6 out]
        n89 = local read "golpi"() -> (w113:T1)
        n90 = call "golpi_mpc_get_access.vi"("don't query version (true)"=TRUE, "allow octave start (true)"=FALSE, "golpi session ref"=w113) -> ("error out"=w121:errorcluster, "GOLPI ref out"=w116:T68, "golpi session out"=w115:T70, "golpi session ref out (copy)"=w118:T1)  [unwired: 3 in, 2 out]
        n91 = Unbundle By Name(w115) -> ("exit command"=w114:string)
        n92 = call "golpi_mpc_close_octave.vi"("exit command (empty)"=w114, "error in"=w121, "GOLPI ref in"=w116) -> ("error out"=w120:errorcluster, "GOLPI ref out (empty)"=w119:T68)  [unwired: 6 in, 1 out]
        n93 = call "golpi_mpc_release.vi"("error in"=w120, "golpi ref or golpi session in"=w119, "golpi session ref"=w118) -> ("error out"=w117:errorcluster)  [unwired: 7 in, 1 out]
        n94 = local write "error out"(w117) -> ()
        n95 = Unbundle By Name(w117) -> ("status"=w122:bool)
        n96 = local write "status"(w122) -> ()
      }
    }
  }
  n97 = call "align_vi_panel.vi"() -> ()  [unwired: 11 in, 1 out]
  n98 = flat-sequence {
    tunnel: w3 -> [_]
    tunnel: w1 -> [w123]
    frame #0 {
      n99 = call "SGUI Register Controls.vi"("register mode (overwrite)"=SGUI_Assign_References_Mode."Release ID", "controls ID (empty)"=w123) -> ("error out"=w125:errorcluster)  [unwired: 15 in, 2 out]
      n100 = call <vilib>:"Clear Errors.vi"("error in (no error)"=w125) -> ()  [unwired: 5 in, 2 out]
    }
  }
  "error out" <- "error in"
  "session out" <- "session in"
